vi "Add Remove Test.vi"() -> ()   [LabVIEW 2013, in "User Control Module Test.lvlib"]
uses:
  User Control Module Test.lvlib
  <vilib>/NI/Tag Bus Module Framework/channel/TBM channel.lvclass
  <vilib>/NI/Tag Bus/tag/Data Type.ctl
  <vilib>/NI/Tag Bus Module Framework/channel/channel classification.ctl
  module/configuration/user control module configuration.lvclass
  <vilib>/NI/Tag Bus/tag/tag descriptor.lvclass
panel:
  out "Deleted Line 2":T1
  out "Deleted Line":string
  out "Success Delete":bool
  out "error out":errorcluster
  out "Success ADD":bool
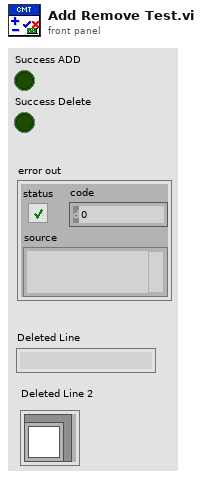
[diagram p1: front panel]
types:
  T1 = cluster{"channel":refnum<class "TBM channel.lvclass">}
  T2 = typedef "TBM channel.lvclass/channel classification.ctl" = enum16{"input data", "output data", "processing parameter", "processing result"}
  T3 = typedef "tag bus.lvlib/tag descriptor.lvclass/Data Type.ctl" = enum16{"Double", "Single", "I64", "I32", "I16", "I8", "U64", "U32", "U16", "U8", "Boolean", "String", "Array of Double", "Array of Single", "Array of I64", "Array of I32", "Array of I16", "Array of I8", "Array of U64", "Array of U32", "Array of U16", "Array of U8", "Array of Boolean", "Array of String"}
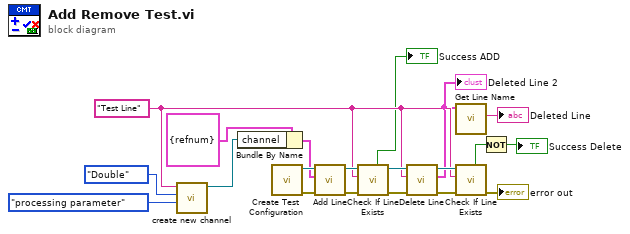
[diagram p0: block diagram]
diagram:
  w7 = "Test Line" ("channel name")
  n1 = call <vilib>:"create new channel.vi"("channel classification"=channel_classification."processing parameter", "data type"=Data_Type."Double", "channel name"=w7) -> ("channel"=w17:refnum<class "TBM channel.lvclass">)  [unwired: 8 in]
  n2 = Bundle By Name(cluster=T1 {"channel"=refnum} ("Line"), "channel"=w17) -> (w8:T1)
  n3 = call "Create Test Configuration.vi"() -> ("error out"=w13:errorcluster, "Module"=w9:refnum<class "user control module configuration.lvclass">)  [unwired: 6 in, 4 out]
  n4 = call-dynamic "Add Line.vi"("error in (no error)"=w13, "Line"=w8, "user control module configuration in"=w9) -> ("error out"=w14:errorcluster, "user control module configuration out"=w12:refnum<class "user control module configuration.lvclass">)  [unwired: 7 in]
  n5 = call-dynamic "Check If Line Exists.vi"("error in (no error)"=w14, "name to locate"=w7, "user control module configuration in"=w12) -> ("error out"=w15:errorcluster, "user control module configuration out"=w11:refnum<class "user control module configuration.lvclass">, "found?"=→"Success ADD":bool)  [unwired: 4 in, 2 out]
  n6 = call-dynamic "Delete Line.vi"("error in"=w15, "Active Line Name"=w7, "user control module configuration in"=w11) -> ("error out"=w16:errorcluster, "Deleted Line"=w4:T1, "user control module configuration out"=w10:refnum<class "user control module configuration.lvclass">)  [unwired: 6 in]
  "Deleted Line 2" <- w4
  n7 = call "Get Line Name.vi"("Line in"=w4) -> ("Name"=→"Deleted Line":string)  [unwired: 8 in, 2 out]
  n8 = call-dynamic "Check If Line Exists.vi"("error in (no error)"=w16, "name to locate"=w7, "user control module configuration in"=w10) -> ("error out"=→"error out":errorcluster, "found?"=w1:bool)  [unwired: 4 in, 3 out]
  n9 = Not(x=w1) -> (.not. x?=→"Success Delete":bool)
